vi "PV ActiveLine - LoggerControlMode.vi"(0 "Referenz in":refnum<visa-resource-name>, 1 "W/R":bool, 5 "logger command":u8(ring) items=["stop", "start", "clear"], 7 "recording interval":u8(ring) items=["1 s", "20 s", "30 s", "1 min", "value change of > 5%", "value change of >10%"], 9 "decimal separator":i8(ring) items=[", (comma)", ". (full stop)"], 11 "Fehler (Eingang)":errorcluster, 12 "Filename":string) -> (4 "Referenz out":refnum<visa-resource-name>, 6 "logger status":i8(ring) items=["stopped", "running"], 8 "recording interval out":i8(ring) items=["1 s", "20 s", "30 s", "1 min", "value change of > 5%", "value change of >10%"], 10 "decimal separator out":i8(ring) items=[", (comma)", ". (full stop)"], 14 "Filename out":string, 15 "Cluster (Ausgang)":errorcluster)   [LabVIEW 2013, in "PV ActiveLine.lvlib"]
doc: "LCM - Start / Stop Data Logger\n\nTransmit: LCM [,a,b,c,ddddddd]\nReceive: a,b,c,ddddddd\n\nData logger command,\na =\n0 .> Stop / data logging stopped\n1 .> Start / data logging started\n2 .> Clear / deletion of measurement data file\n(ending CSV) from USB memory stick\n\nData logging interval,\nb =\n0 .> Logging interval 1/s\n1 .> Logging interval 1/10 s\n2 .> Logging interval 1/30 s\n3 .> Logging interval 1/60 s\n4 .> Logging interval in the event of measurement\nvalue changes .1% s\n5 .> Logging interval in the event of measurement\nvalue changes .5% s\n\nDecimal separator,\nc =\n0 .> , (decimal comma)\n1 .> . (decimal point)\n\nFile name (max. 7 digits)\nddddddd"
uses:
  <instrlib>/PV ActiveLine/PV ActiveLine.lvlib
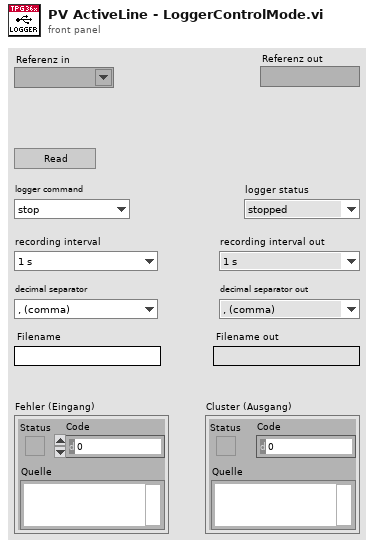
[diagram p1: front panel]
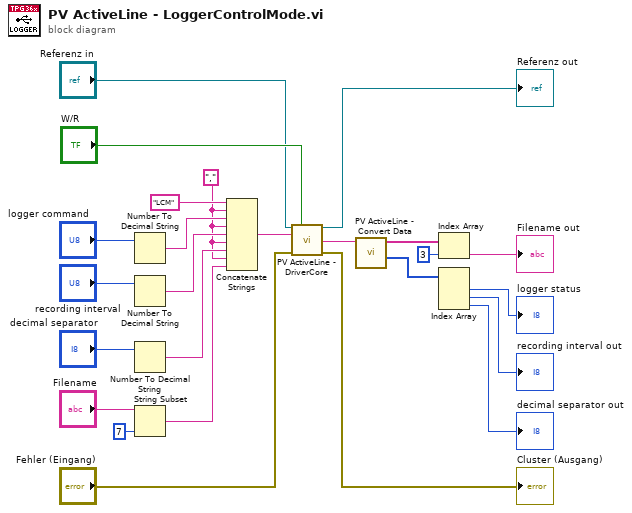
[diagram p0: block diagram]
diagram:
  w9 = "," ("string")
  n1 = Number To Decimal String(number="logger command") -> (decimal integer string=w22:string)  [unwired: 1 in]
  n2 = Number To Decimal String(number="recording interval") -> (decimal integer string=w18:string)  [unwired: 1 in]
  n3 = Number To Decimal String(number="decimal separator") -> (decimal integer string=w12:string)  [unwired: 1 in]
  n4 = String Subset(string="Filename", length (rest)=7 ("length (rest)")) -> (substring=w14:string)  [unwired: 1 in]
  n5 = Concatenate Strings("LCM", w9, w22, w9, w18, w9, w12, w9, w14) -> (w23:string)
  n6 = call <instrlib>:"PV ActiveLine - DriverCore.vi"("Referenz in"="Referenz in", "Write/Read"="W/R", "Command"=w23, "Fehler (Eingang)"="Fehler (Eingang)") -> ("Referenz out"=→"Referenz out":refnum<visa-resource-name>, "String Out"=w8:string, "Cluster (Ausgang)"=→"Cluster (Ausgang)":errorcluster)  [unwired: 9 in]
  n7 = call <instrlib>:"PV ActiveLine - Convert Data.vi"("String in"=w8) -> ("Integer Out"=w4:i32[], "String out"=w7:string[])  [unwired: 7 in, 2 out]
  n8 = Index Array(array=w7, index=3 ("Index")) -> (element=→"Filename out":string)
  n9 = Index Array(array=w4) -> (element #1=→"logger status":i32, element #2=→"recording interval out":i32, element #3=→"decimal separator out":i32)  [unwired: 3 in]
